vi "Get next waypoint.vi"(11 "Waypoint Array In":T2(array[cluster]) {"Time"."GPS Time of Week" format="%.3f"; "Velocity, Correction & SET"."Extended Navigation Mode" items=["Non Differential"=0, "Code (RTCM Type 1 & 9)"=1, "Code, Single Frequency (WAAS)"=2, "Code, Dual Frequency (WAAS)"=3, "Code, Single Frequency (WCT)"=4, "Code/RCP, Dual Frequency (WCT)"=5, "Code, Single Frequency (RTG)"=6, "Code (RTCM Type 1 & 9) Dual Frequency"=10, "Code/RCP, Dual Frequency (RTG)"=11, "Code, Single Frequency (NCT-RTK)"=12, "Code, Single Frequency (RTCM 18 & 19)"=13, "Code, Single Frequency (RTCM 21 & 22)"=14, "Code, Single Frequency (CMR)"=15, "Code, Dual Frequency (NCT-RTK)"=16, "Code, Dual Frequency (RTCM 18 & 19)"=17, "Code, Dual Frequency (RTCM 20 & 21)"=18, "Code, Dual Frequency (CMR)"=19, "RTK (NCT-RTK)"=20, "RTK (RTCM 18 & 19)"=21, "RTK (RTCM 20 & 21)"=22, "RTK (CMR)"=23, "Code, Single Frequency with SET (RTG)"=24, "Code/RCP, Dual Frequency with SET (RTG)"=25, "RTK Extend"=26]}) -> (1 "No more waypoints":bool, 2 "Next Waypoint":T1, 3 "Waypoint Array Out":T2(array[cluster]))   [LabVIEW 2011]
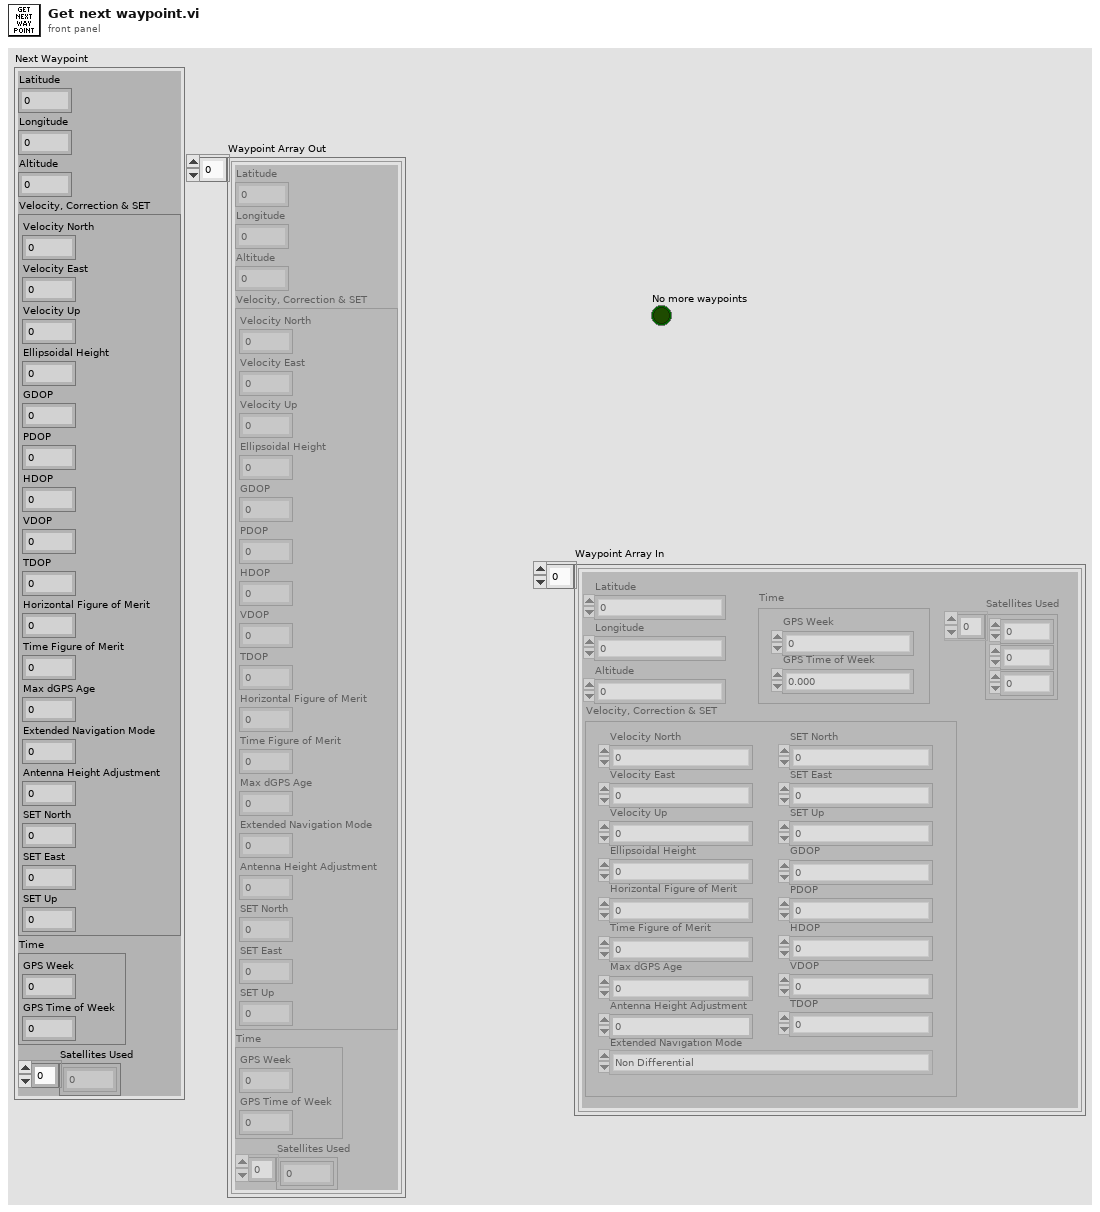
[diagram p1: front panel]
types:
  T1 = cluster{"Latitude":dbl, "Longitude":dbl, "Altitude":dbl, "Velocity, Correction & SET":cluster{"Velocity North":dbl, "Velocity East":dbl, "Velocity Up":dbl, "Ellipsoidal Height":dbl, "GDOP":sgl, "PDOP":sgl, "HDOP":sgl, "VDOP":sgl, "TDOP":sgl, "Horizontal Figure of Merit":u8, "Time Figure of Merit":u8, "Max dGPS Age":sgl, "Extended Navigation Mode":u8, "Antenna Height Adjustment ":dbl, "SET North":i32, "SET East":i32, "SET Up":i32}, "Time":cluster{"GPS Week":u16, "GPS Time of Week":sgl}, "Satellites Used":i32[]}
  T2 = cluster{"Latitude":dbl, "Longitude":dbl, "Altitude":dbl, "Velocity, Correction & SET":cluster{"Velocity North":dbl, "Velocity East":dbl, "Velocity Up":dbl, "Ellipsoidal Height":dbl, "GDOP":sgl, "PDOP":sgl, "HDOP":sgl, "VDOP":sgl, "TDOP":sgl, "Horizontal Figure of Merit":u8, "Time Figure of Merit":u8, "Max dGPS Age":sgl, "Extended Navigation Mode":u8, "Antenna Height Adjustment ":dbl, "SET North":i32, "SET East":i32, "SET Up":i32}, "Time":cluster{"GPS Week":u16, "GPS Time of Week":sgl}, "Satellites Used":i32[]}[]
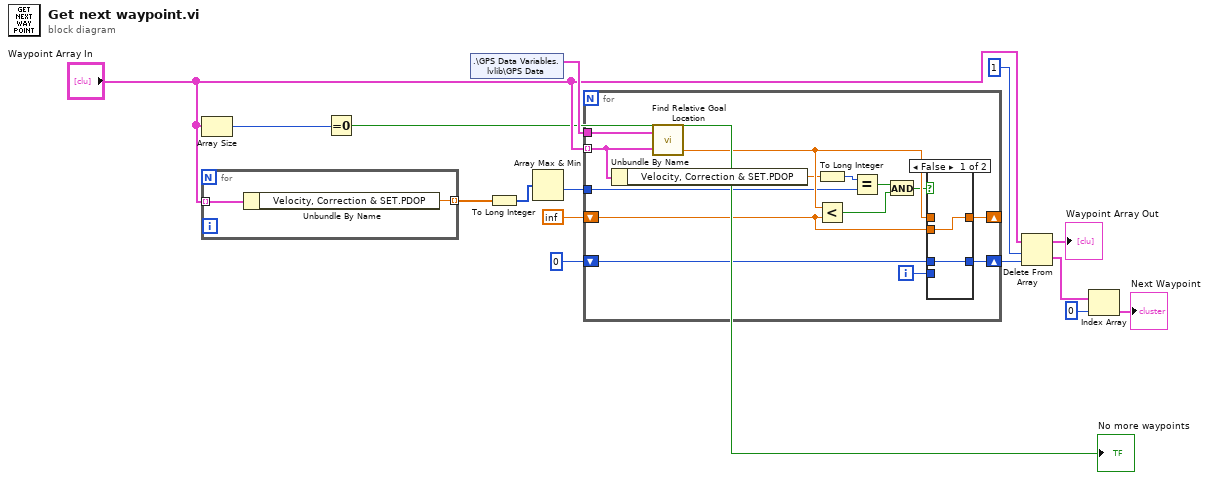
[diagram p0: block diagram]
diagram:
  n1 = Array Size(array="Waypoint Array In") -> (size(s)=w7:i32)
  n2 = for {
    tunnel: "Waypoint Array In" -> [w17] mode=indexing
    tunnel: [w16] -> w2 mode=indexing
    n3 = Unbundle By Name(w17) -> ("Velocity, Correction & SET.PDOP"=w16:sgl)
  }
  n4 = Equal To 0?(x=w7) -> (x = 0?=→"No more waypoints":bool)
  n5 = shared-variable ".\\GPS Data Variables.lvlib\\GPS Data"() -> (w15:T1)  [unwired: 1 in, 1 out]
  n6 = To Long Integer(number=w2) -> (32bit integer=w1:i32[])
  n7 = Array Max & Min(array=w1) -> (min value=w9:i32)  [unwired: 3 out]
  n8 = for {
    tunnel: w15 -> [w31]
    shift-right: [w26] -> _
    shift-left: inf -> [w27]
    shift-right: [w29] -> w11
    shift-left: 0 -> [w28]
    tunnel: "Waypoint Array In" -> [w23] mode=indexing
    tunnel: w9 -> [w24]
    i -> [w30]
    n9 = Unbundle By Name(w23) -> ("Velocity, Correction & SET.PDOP"=w19:sgl)
    n10 = call "Find Relative Goal Location.vi"("Current Position"=w31, "Goal Position"=w23) -> ("Target Distance"=w25:dbl)  [unwired: 2 out]
    n11 = To Long Integer(number=w19) -> (32bit integer=w18:i32)
    n12 = Less?(x=w25, y=w27) -> (x < y?=w21:bool)
    n13 = Equal?(x=w18, y=w24) -> (x = y?=w22:bool)
    n14 = And(x=w22, y=w21) -> (x .and. y?=w20:bool)
    n15 = case shown="False" w20 {
      tunnel: w30 -> [_ w35]
      tunnel: [w33 w35] -> w29
      tunnel: w28 -> [w33 _]
      tunnel: w27 -> [w32 _]
      tunnel: [w32 w34] -> w26
      tunnel: w25 -> [_ w34]
      frame False {
      }
      frame True {
      }
    }
  }
  n16 = Delete From Array(array="Waypoint Array In", length=1, index=w11) -> (deleted portion=w5:T2, array with subset deleted=→"Waypoint Array Out":T2)
  n17 = Index Array(array=w5, index=0) -> (element=→"Next Waypoint":T1)
